vi "Control_Rack_Controler.vi"(0 "Times":dbl[](array[numeric]), 1 "Voltages Toroidal (Keep below |10|)":dbl[](array[numeric]), 2 "Voltages Helical (Keep below |10|)":dbl[](array[numeric]), 3 "error out":errorcluster, 4 "Data in":T2) -> (5 "error out 2":errorcluster, 6 "Data out":T2)   [LabVIEW 2017]
uses:
  Type_Defs/Data.ctl
  Type_Defs/Diagnostics.ctl
  Type_Defs/Systems.ctl
  <vilib>/DAQmx/write.llb/DAQmx Write (Analog DBL 1Chan 1Samp).vi
  <vilib>/DAQmx/create/channels.llb/DAQmx Create Channel (AO-Voltage-Basic).vi
  <vilib>/DAQmx/miscellaneous.llb/DAQmx Fill In Error Info.vi
  <vilib>/express/express shared/transition.llb/Dynamic To Waveform Array.vi
  <vilib>/express/express signal manip/GetorSetDDTAttributes/Set DDT Attributes/SetT0.vi
  <vilib>/express/express shared/transition.llb/Waveform Array To Dynamic.vi
  <vilib>/express/express signal manip/GetorSetDDTAttributes/Set DDT Attributes/Set DDT Properties.xnode
panel:
  out "Toroidal Limited Current Set Point":dbl(graph)=-0.021820068359375
  out "Torroidal Voltage Feedback":dbl(graph)=-0.021820068359375
  out "Torroidal Current Feedback":dbl(graph)=-0.021820068359375
  out "Helix Current Feedback":dbl(graph)=-0.021820068359375
  out "Helix Voltage Feedback":dbl(graph)=-0.021820068359375
  out "Helix Limited Current Set Point":dbl(graph)=-0.021820068359375
  out "Experiment State":T1(ring)
  out "Experiment Purpose":string
  out "Start Time":timestamp
  out "Shot Number":i32
  out "Operator":string
  out "Running":bool
  out "Voltage Toroidal":dbl
  out "Time":i64
  out "Voltage Helical":dbl
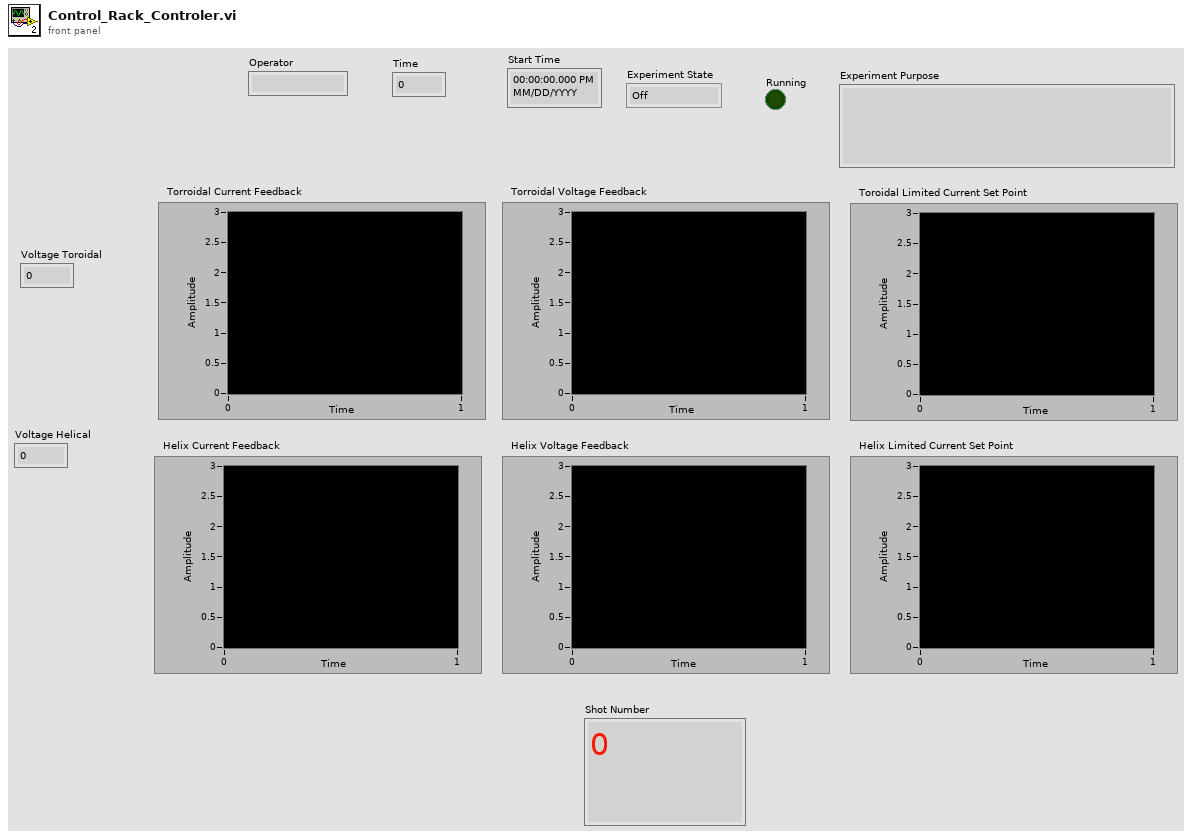
[diagram p1: front panel]
types:
  T1 = enum16{"Off", "Setting Up", "Ready", "In Progress", "Shutting Down"}
  T2 = typedef "Data.ctl" = cluster{"User Name":string, "Experiment Number":i32, "Start Time":timestamp, "Data":dbl[], "Step Number":i32, "Step Instructions":string, "Diagnostics":T3, "Experiment Purpose":string, "Experiment State":enum16{"Off", "Setting Up", "Ready", "In Progress", "Shutting Down"}, "Systems":T4, "Vacuum Pressure":dbl, "Fieldpoints":cluster{"System Boolean Fieldpoints":cluster{"Compressed Air":refnum<k21>, "T-20kV Power Switch":refnum<k21>, "T-Rectifier":refnum<k21>, "Engage Interlock":refnum<k21>, "Ventilator":refnum<k21>, "Magnetron":refnum<k21>, "H-20kV Power Switch":refnum<k21>, "H-Rectifier":refnum<k21>, "Main Water Pump":refnum<k21>, "WEGA Water Pump":refnum<k21>, "Gas Inlet Valves":refnum<k21>}, "Step Fieldpoints":cluster{"Exhaust Ventillator":refnum<k21>, "Compressed Air":refnum<k21>, "Water Pressure":refnum<k21>, "Interlock":refnum<k21>, "Toroidal Power Supply 1":refnum<k21>, "Toroidal Power Supply 2":refnum<k21>, "Toroidal Rectifier":refnum<k21>, "Helical Power Supply":refnum<k21>, "Helical Rectifier":refnum<k21>, "6kW Magnetron Standby":refnum<k21>, "20kW Magnetron Standby":refnum<k21>}}, "Pressure History":cluster{"Seconds into Experiment":i32[], "Pressure Data":dbl[]}, "Time Computer Control":dbl[], "Toroidal Voltage Computer Control":dbl[], "Helical Voltage Computer Control":dbl[], "Toroidal Current":dbl[], "Toroidal Voltage":dbl[], "Toroidal Current Set Point":dbl[], "Helical Current Set Point":dbl[], "Helical Voltage":dbl[], "Helical Current":dbl[], "Experiment Folder":path, "Run Another Shot?":bool}
  T3 = typedef "Diagnostics.ctl" = cluster{"Langmuir Probe":bool, "Rogowski 1":bool, "Rogowski 2":bool, "Rogowski 3":bool, "B-dot 1":bool, "B-dot 2":bool}
  T4 = typedef "Systems.ctl" = cluster{"Compressed Air":bool, "T-20kV Power Switch":bool, "T-Rectifier":bool, "Engage Interlock":bool, "Ventilator":bool, "Magnetron":bool, "H-20kV Power Switch":bool, "H-Rectifier":bool, "Main Water Pump":bool, "WEGA Water Pump":bool, "Gas Inlet Valves":bool}
  T5 = enum32{"Invalid", "Standard", "Closed", "Hidden", "Minimized", "Maximized"}
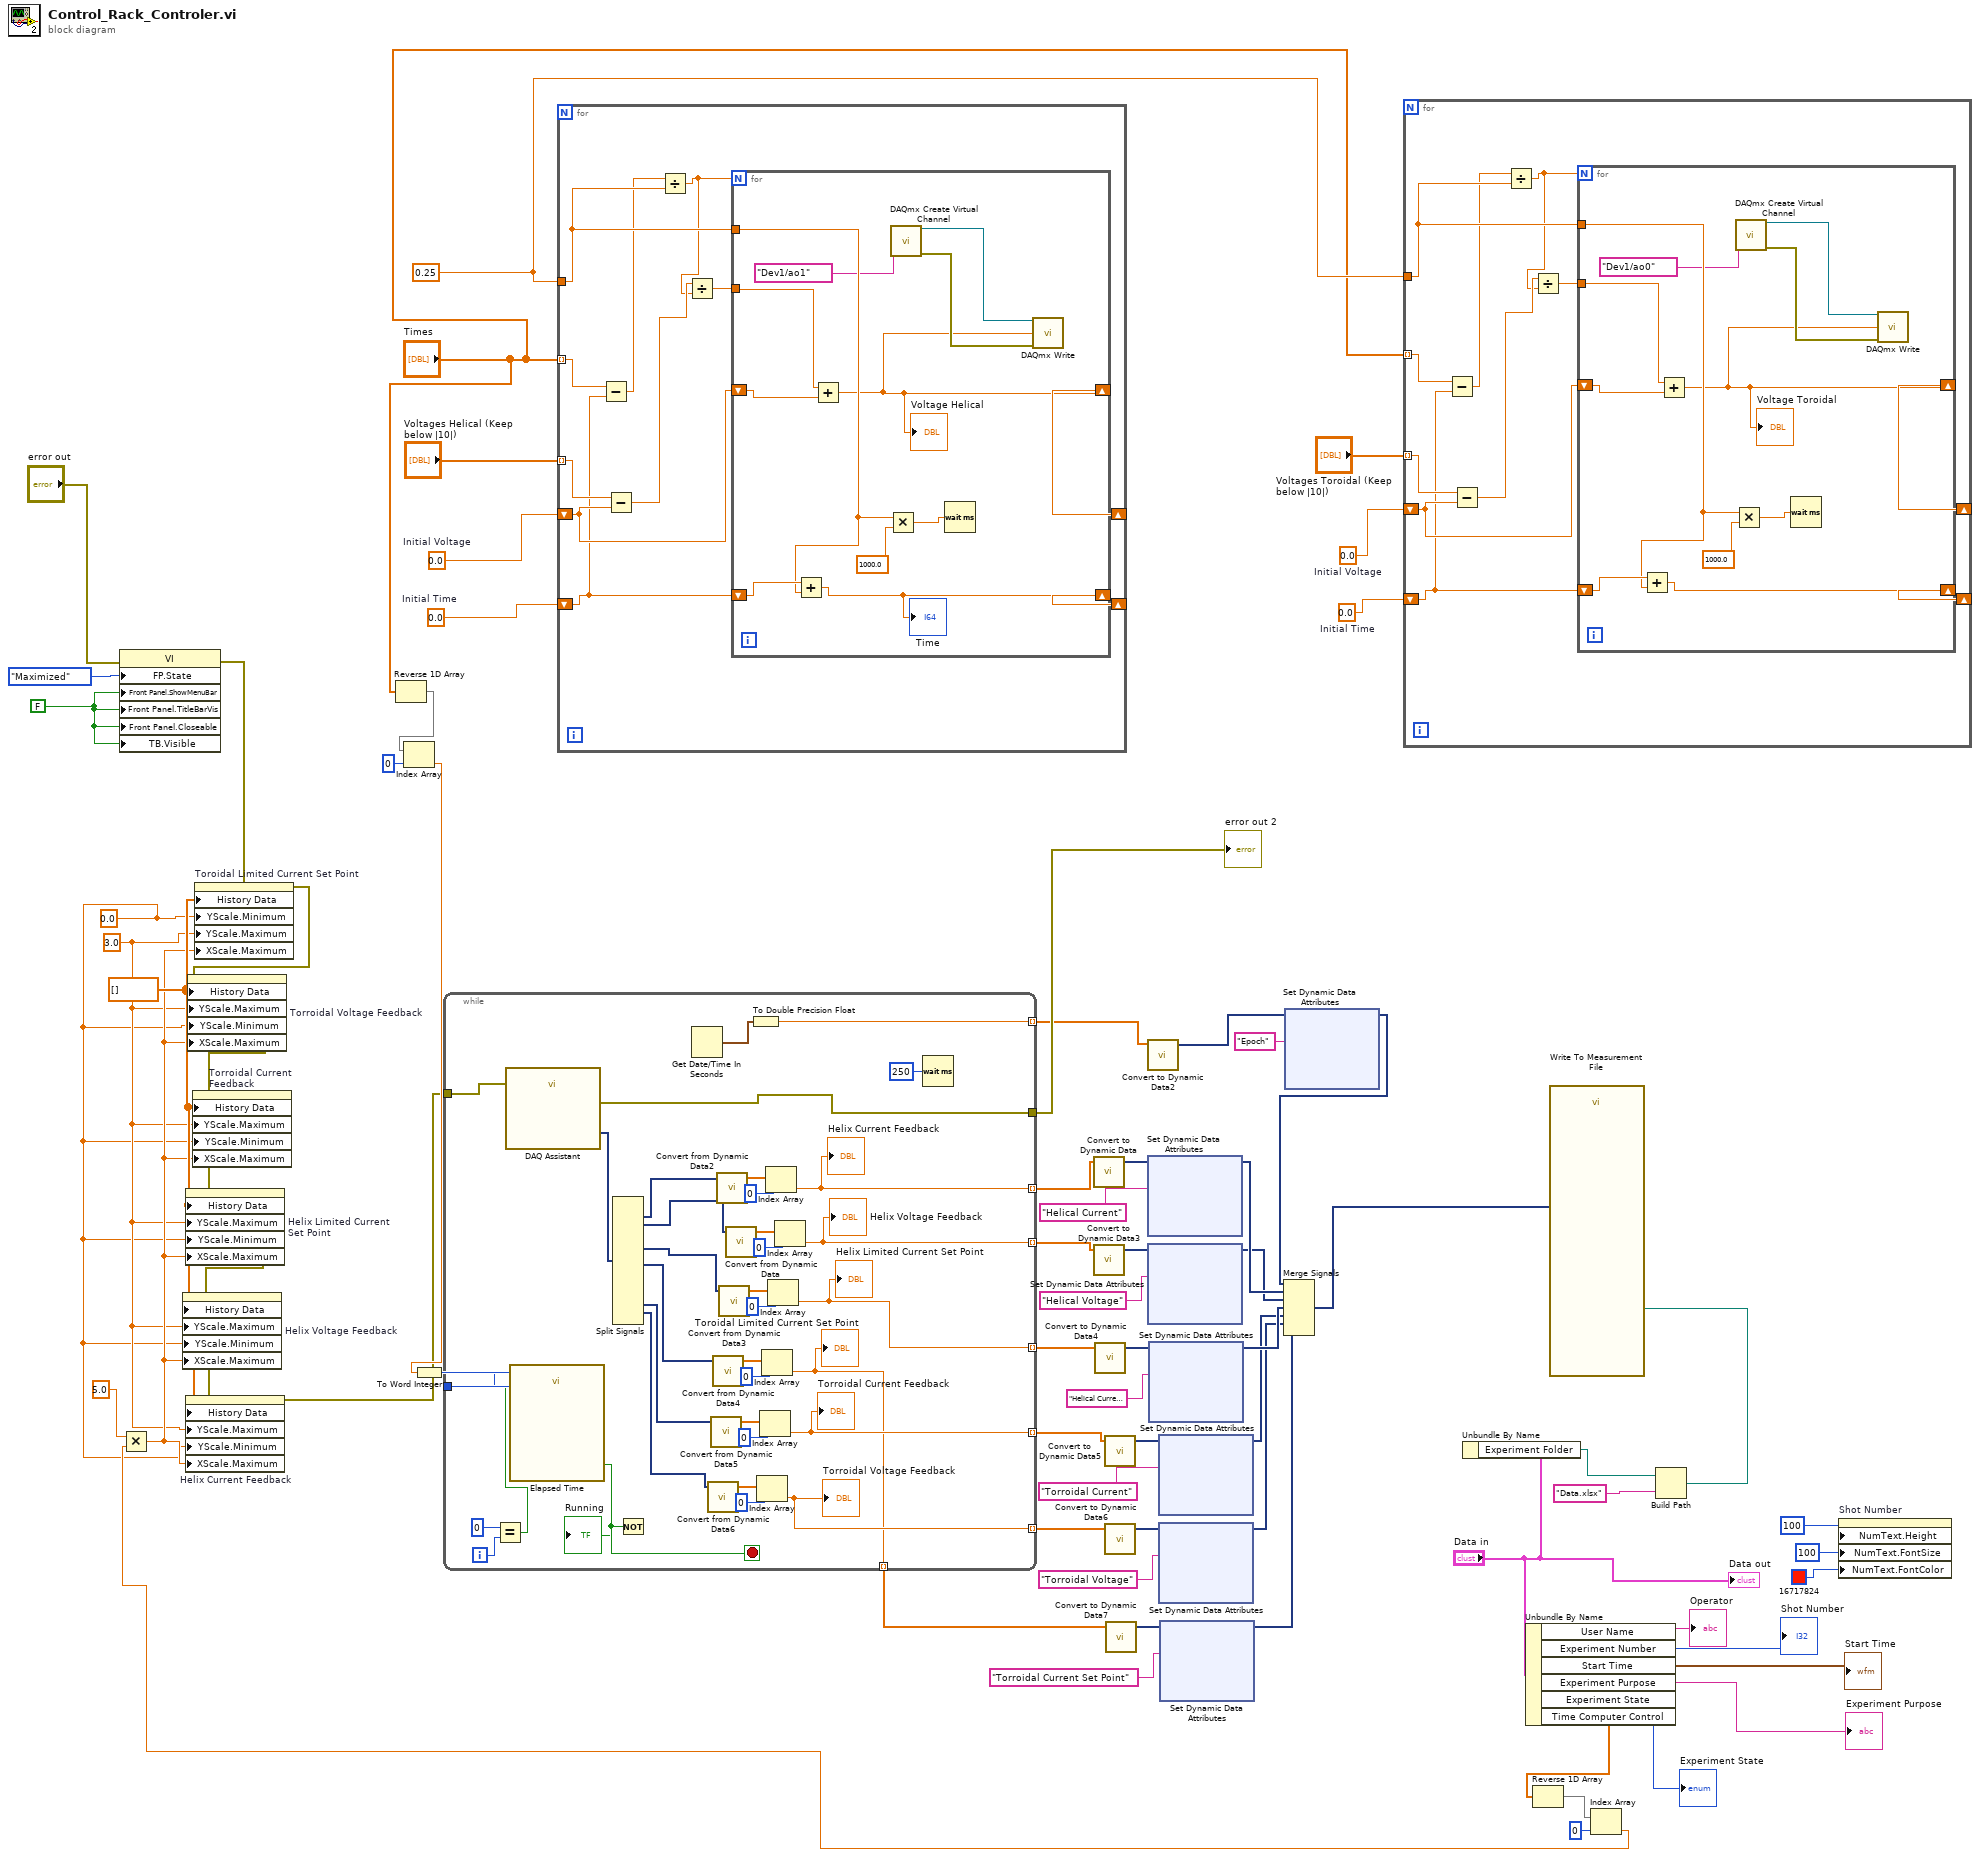
[diagram p0: block diagram]
diagram:
  w1 = FALSE ("Front Panel Window:Show Menu Bar")
  w9 = 3.0 ("Y Scale.Range:Maximum")
  w8 = 0.0 ("Y Scale.Range:Minimum")
  w14 = dbl[] [] ("History Data")
  w67 = 0.25 ("Timestep (in seconds, keep above 1/20s)")
  w70 = 0.0  # Initial Time
  w69 = 0.0  # Initial Voltage
  w71 = 0.0  # Initial Time
  w72 = 0.0  # Initial Voltage
  n1 = property class="VI"(error in="error out", "FP.State"=T5."Maximized" ("Front Panel Window:State"), "Front Panel.ShowMenuBar"=w1, "Front Panel.TitleBarVis"=w1, "Front Panel.Closeable"=w1, "TB.Visible"=w1) -> (error out=w3:errorcluster)  [unwired: 1 in, 1 out]
  n2 = Reverse 1D Array(array="Times") -> (reversed array=w65:dbl[])
  n3 = Index Array(array=w65, index=0) -> (element=w62:dbl)
  n4 = To Word Integer(number=w62) -> (16bit integer=w61:i16)
  n5 = for {
    tunnel: "Voltages Helical (Keep below |10|)" -> [w84] mode=indexing
    tunnel: "Times" -> [w77] mode=indexing
    tunnel: w67 -> [w79]
    shift-right: [w80] -> _
    shift-left: w72 -> [w83]
    shift-right: [w78] -> _
    shift-left: w71 -> [w76]
    n6 = Subtract(x=w77, y=w76) -> (x-y=w75:dbl)
    n7 = Subtract(x=w84, y=w83) -> (x-y=w82:dbl)
    n8 = Divide(x=w75, y=w79) -> (x/y=w74:dbl)
    n9 = Divide(x=w82, y=w74) -> (x/y=w81:dbl)
    n10 = for {
      N: w74 -> [_]
      shift-right: [w85] -> w80
      shift-left: w83 -> [w95]
      tunnel: w81 -> [w94]
      tunnel: w79 -> [w91]
      shift-right: [w89] -> w78
      shift-left: w76 -> [w93]
      n11 = Add(x=w93, y=w91) -> (x+y=w89:dbl)
      "Time" <- w89
      n12 = Add(x=w94, y=w95) -> (x+y=w85:dbl)
      "Voltage Helical" <- w85
      n13 = Multiply(x=w91, y=1000.0) -> (x*y=w92:dbl)
      n14 = call-poly <vilib>:"DAQmx Create Virtual Channel.vi"("physical channels"=tag "Dev1/ao1" ("write channel (torr = ao0, hel = ao1)")) -> ("task out"=w86:refnum<k21>, "error out"=w87:errorcluster)  [unwired: 13 in]
      n15 = Wait (ms)(milliseconds to wait=w92) -> ()  [unwired: 1 out]
      n16 = call-poly <vilib>:"DAQmx Write.vi"("task/channels in"=w86, "data"=w85, "error in"=w87) -> ()  [unwired: 10 in, 3 out]
    }
  }
  n17 = for {
    tunnel: "Voltages Toroidal (Keep below |10|)" -> [w106] mode=indexing
    tunnel: "Times" -> [w99] mode=indexing
    tunnel: w67 -> [w101]
    shift-right: [w102] -> _
    shift-left: w69 -> [w105]
    shift-right: [w100] -> _
    shift-left: w70 -> [w98]
    n18 = Subtract(x=w99, y=w98) -> (x-y=w97:dbl)
    n19 = Subtract(x=w106, y=w105) -> (x-y=w104:dbl)
    n20 = Divide(x=w97, y=w101) -> (x/y=w96:dbl)
    n21 = Divide(x=w104, y=w96) -> (x/y=w103:dbl)
    n22 = for {
      N: w96 -> [_]
      shift-right: [w107] -> w102
      shift-left: w105 -> [w117]
      tunnel: w103 -> [w116]
      tunnel: w101 -> [w113]
      shift-right: [w111] -> w100
      shift-left: w98 -> [w115]
      n23 = Add(x=w115, y=w113) -> (x+y=w111:dbl)
      n24 = Add(x=w116, y=w117) -> (x+y=w107:dbl)
      "Voltage Toroidal" <- w107
      n25 = Multiply(x=w113, y=1000.0) -> (x*y=w114:dbl)
      n26 = call-poly <vilib>:"DAQmx Create Virtual Channel.vi"("physical channels"=tag "Dev1/ao0" ("write channel (torr = ao0, hel = ao1) 2")) -> ("task out"=w108:refnum<k21>, "error out"=w109:errorcluster)  [unwired: 13 in]
      n27 = Wait (ms)(milliseconds to wait=w114) -> ()  [unwired: 1 out]
      n28 = call-poly <vilib>:"DAQmx Write.vi"("task/channels in"=w108, "data"=w107, "error in"=w109) -> ()  [unwired: 10 in, 3 out]
    }
  }
  n29 = Unbundle By Name("Data in") -> ("Experiment Folder"=w59:path)
  n30 = Unbundle By Name("Data in") -> ("User Name"=→"Operator":string, "Experiment Number"=→"Shot Number":i32, "Start Time"=→"Start Time":timestamp, "Experiment Purpose"=→"Experiment Purpose":string, "Experiment State"=→"Experiment State":T1, "Time Computer Control"=w17:dbl[])
  n31 = Reverse 1D Array(array=w17) -> (reversed array=w16:dbl[])
  n32 = Index Array(array=w16, index=0) -> (element=w11:dbl)
  n33 = Multiply(x=5.0, y=w11) -> (x*y=w10:dbl)
  n34 = property on="Toroidal Limited Current Set Point" class="WFChart (strict)"(error in=w3, "History Data"=w14, "YScale.Minimum"=w8, "YScale.Maximum"=w9, "XScale.Maximum"=w10) -> (error out=w13:errorcluster)  [unwired: 1 in, 1 out]
  n35 = property on="Torroidal Voltage Feedback" class="WFChart (strict)"(error in=w13, "History Data"=w14, "YScale.Maximum"=w9, "YScale.Minimum"=w8, "XScale.Maximum"=w10) -> (error out=w22:errorcluster)  [unwired: 1 in, 1 out]
  n36 = property on="Torroidal Current Feedback" class="WFChart (strict)"(error in=w22, "History Data"=w14, "YScale.Maximum"=w9, "YScale.Minimum"=w8, "XScale.Maximum"=w10) -> (error out=w21:errorcluster)  [unwired: 1 in, 1 out]
  n37 = property on="Helix Limited Current Set Point" class="WFChart (strict)"(error in=w21, "History Data"=w14, "YScale.Maximum"=w9, "YScale.Minimum"=w8, "XScale.Maximum"=w10) -> (error out=w20:errorcluster)  [unwired: 1 in, 1 out]
  n38 = property on="Helix Voltage Feedback" class="WFChart (strict)"(error in=w20, "History Data"=w14, "YScale.Maximum"=w9, "YScale.Minimum"=w8, "XScale.Maximum"=w10) -> (error out=w19:errorcluster)  [unwired: 1 in, 1 out]
  n39 = property on="Helix Current Feedback" class="WFChart (strict)"(error in=w19, "History Data"=w14, "YScale.Maximum"=w9, "YScale.Minimum"=w8, "XScale.Maximum"=w10) -> (error out=w18:errorcluster)  [unwired: 1 in, 1 out]
  n40 = while {
    tunnel: [w126] -> w63
    tunnel: w61 -> [w152]
    tunnel: [w121] -> w25 mode=indexing
    tunnel: [w122] -> w36 mode=indexing
    tunnel: [w125] -> w35 mode=indexing
    tunnel: [w123] -> w34 mode=indexing
    tunnel: [w124] -> w33 mode=indexing
    tunnel: [w119] -> w32 mode=indexing
    tunnel: [w128] -> w24 mode=indexing
    tunnel: w18 -> [w120]
    i -> [w127]
    stop <- w131 stop-if-true
    n41 = Equal?(x=0, y=w127) -> (x = y?=w132:bool)
    n42 = call "DAQ Assistant"("error in"=w120) -> ("data"=w153:dynamicdata, "error out"=w126:errorcluster)  [unwired: 16 in, 1 out]
    n43 = call "Elapsed Time"("Time Target (s)"=w152, "Reset"=w132) -> ("Time has Elapsed"=w131:bool)  [unwired: 10 in, 7 out]
    n44 = Split Signals(w153) -> (w151:dynamicdata, w138:dynamicdata, w137:dynamicdata, w136:dynamicdata, w135:dynamicdata, w134:dynamicdata)  [unwired: 16 in, 10 out]
    n45 = Not(x=w131) -> (.not. x?=→"Running":bool)
    n46 = Get Date/Time In Seconds() -> (seconds since 1Jan1904=w129:timestamp)
    n47 = call "Convert from Dynamic Data6"("Dynamic Data Type"=w134) -> ("Array"=w140:dbl[])  [unwired: 3 in]
    n48 = call "Convert from Dynamic Data5"("Dynamic Data Type"=w135) -> ("Array"=w142:dbl[])  [unwired: 3 in]
    n49 = call "Convert from Dynamic Data4"("Dynamic Data Type"=w136) -> ("Array"=w144:dbl[])  [unwired: 3 in]
    n50 = call "Convert from Dynamic Data2"("Dynamic Data Type"=w151) -> ("Array"=w150:dbl[])  [unwired: 3 in]
    n51 = call "Convert from Dynamic Data3"("Dynamic Data Type"=w137) -> ("Array"=w146:dbl[])  [unwired: 3 in]
    n52 = call "Convert from Dynamic Data"("Dynamic Data Type"=w138) -> ("Array"=w148:dbl[])  [unwired: 3 in]
    n53 = To Double Precision Float(number=w129) -> (double precision float=w128:dbl)
    n54 = Index Array(array=w140, index=0) -> (element=w124:dbl)
    "Torroidal Voltage Feedback" <- w124
    n55 = Index Array(array=w142, index=0) -> (element=w123:dbl)
    "Torroidal Current Feedback" <- w123
    n56 = Index Array(array=w144, index=0) -> (element=w119:dbl)
    "Toroidal Limited Current Set Point" <- w119
    n57 = Index Array(array=w150, index=0) -> (element=w121:dbl)
    "Helix Current Feedback" <- w121
    n58 = Index Array(array=w146, index=0) -> (element=w125:dbl)
    "Helix Limited Current Set Point" <- w125
    n59 = Index Array(array=w148, index=0) -> (element=w122:dbl)
    "Helix Voltage Feedback" <- w122
    n60 = Wait (ms)(milliseconds to wait=u32 250) -> ()  [unwired: 1 out]
  }
  "error out 2" <- w63
  n61 = call "Convert to Dynamic Data"("Array"=w25) -> ("Dynamic Data Type"=w57:dynamicdata)  [unwired: 3 in]
  n62 = call "Convert to Dynamic Data3"("Array"=w36) -> ("Dynamic Data Type"=w50:dynamicdata)  [unwired: 3 in]
  n63 = call "Convert to Dynamic Data4"("Array"=w35) -> ("Dynamic Data Type"=w49:dynamicdata)  [unwired: 3 in]
  n64 = call "Convert to Dynamic Data5"("Array"=w34) -> ("Dynamic Data Type"=w48:dynamicdata)  [unwired: 3 in]
  n65 = call "Convert to Dynamic Data6"("Array"=w33) -> ("Dynamic Data Type"=w46:dynamicdata)  [unwired: 3 in]
  n66 = call "Convert to Dynamic Data7"("Array"=w32) -> ("Dynamic Data Type"=w23:dynamicdata)  [unwired: 3 in]
  n67 = call "Convert to Dynamic Data2"("Array"=w24) -> ("Dynamic Data Type"=w55:dynamicdata)  [unwired: 3 in]
  n68 = xnode "Set Dynamic Data Attributes"("Signals In"=w57, "Signal Name"="Helical Current") -> ("Signals Out"=w53:dynamicdata)  [unwired: 2 in, 1 out]
  n69 = xnode "Set Dynamic Data Attributes"("Signals In"=w50, "Signal Name"="Helical Voltage") -> ("Signals Out"=w45:dynamicdata)  [unwired: 2 in, 1 out]
  n70 = xnode "Set Dynamic Data Attributes"("Signals In"=w49, "Signal Name"="Helical Current Set Point") -> ("Signals Out"=w44:dynamicdata)  [unwired: 2 in, 1 out]
  n71 = xnode "Set Dynamic Data Attributes"("Signals In"=w48, "Signal Name"="Torroidal Current") -> ("Signals Out"=w43:dynamicdata)  [unwired: 2 in, 1 out]
  n72 = xnode "Set Dynamic Data Attributes"("Signals In"=w46, "Signal Name"="Torroidal Voltage") -> ("Signals Out"=w42:dynamicdata)  [unwired: 2 in, 1 out]
  n73 = xnode "Set Dynamic Data Attributes"("Signals In"=w23, "Signal Name"="Torroidal Current Set Point") -> ("Signals Out"=w41:dynamicdata)  [unwired: 2 in, 1 out]
  n74 = xnode "Set Dynamic Data Attributes"("Signals In"=w55, "Signal Name"="Epoch") -> ("Signals Out"=w52:dynamicdata)  [unwired: 2 in, 1 out]
  n75 = Merge Signals(w52, w53, w45, w44, w43, w42, w41) -> (w51:dynamicdata)
  n76 = Build Path(base path=w59, name or relative path="Data.xlsx") -> (appended path=w60:path)
  n77 = call "Write To Measurement File"("Signals"=w51, "Filename"=w60) -> ()  [unwired: 15 in, 3 out]
  n78 = property on="Shot Number" class="DigNum (strict)"("NumText.Height"=u32 100 ("Numeric Text.Size:Height"), "NumText.FontSize"=u32 100 ("Numeric Text.Font:Size"), "NumText.FontColor"=u32 16717824) -> ()  [unwired: 2 in, 2 out]
  "Data out" <- "Data in"
